vi "Get Object Metadata.vi"(4 "Region":T1, 6 "Version ID":string, 7 "Request Parameters":T2, 8 "error in (no error)":errorcluster, 9 "Bucket":string, 10 "Object Path":string) -> (0 "error out":errorcluster, 2 "HeadObjectResult":T4)   [LabVIEW 2015, in "LV Interface for Amazon S3.lvlib"]
doc: "This operation <B>retrieves information and metadata associated with an object</B> from Amazon S3. You <B>must have READ access</B> to the object. If you grant READ access to the anonymous user, you can return the object without using an authorization header."
uses:
  LV Interface for Amazon S3.lvlib
  Typedefs/AMZ_S3_API_HEADObjectResult.ctl
  Typedefs/AMZ_S3_API_GETObjectResult.ctl
  Typedefs/AMZ_S3_Key-Value pair.ctl
  Typedefs/AMZ_S3_API_GET Object Request Parameters.ctl
  Typedefs/AMZ_S3_API_GET Request Range.ctl
  Typedefs/AMZ_S3_LocationConstraint.ctl
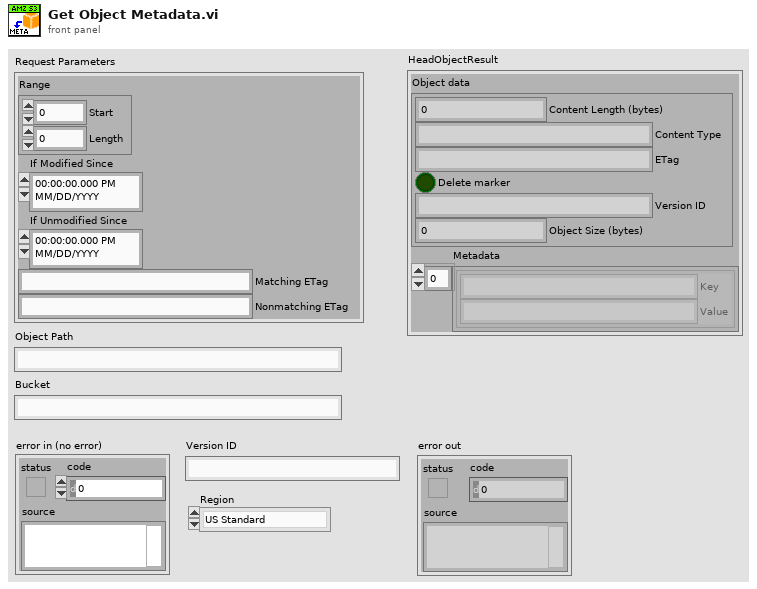
[diagram p1: front panel]
types:
  T1 = typedef "LV Interface for Amazon S3.lvlib/AMZ_S3_LocationConstraint.ctl" = enum16{"US Standard", "us-east-2", "us-west-1", "us-west-2", "ap-northeast-1", "ap-northeast-2", "ap-southeast-1", "ap-southeast-2", "ca-central-1", "eu-central-1", "eu-west-1", "eu-west-2", "sa-east-1"}
  T2 = typedef "LV Interface for Amazon S3.lvlib/AMZ_S3_API_GET Object Request Parameters.ctl" = cluster{"Range":T3, "If Modified Since":timestamp, "If Unmodified Since":timestamp, "Matching ETag":string, "Nonmatching ETag":string}
  T3 = typedef "LV Interface for Amazon S3.lvlib/AMZ_S3_API_GET Request Range.ctl" = cluster{"Start":i64, "Length":i64}
  T4 = typedef "LV Interface for Amazon S3.lvlib/AMZ_S3_API_HEADObjectResult.ctl" = cluster{"Object data":T5, "Metadata":T6[]}
  T5 = typedef "LV Interface for Amazon S3.lvlib/AMZ_S3_API_GETObjectResult.ctl" = cluster{"Content Length (bytes)":u64, "Content Type":string, "ETag":string, "Delete marker":bool, "Version ID":string, "Object Size (bytes)":u64}
  T6 = typedef "LV Interface for Amazon S3.lvlib/AMZ_S3_Key-Value pair.ctl" = cluster{"Key":string, "Value":string}
  T7 = typedef "LV Interface for Amazon S3.lvlib/AMZ_S3_HTTP Header-Value pair.ctl" = cluster{"Header":string, "Value":string}
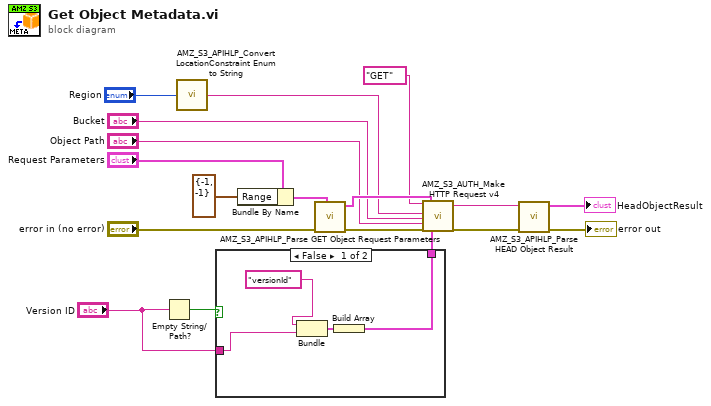
[diagram p0: block diagram]
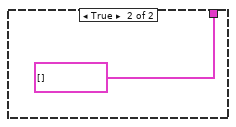
[diagram p2: hidden frame]
diagram:
  n1 = Empty String/Path?(string/path="Version ID") -> (empty?=w5:bool)
  n2 = call "AMZ_S3_APIHLP_Convert LocationConstraint Enum to String.vi"("Location"="Region") -> ("Location String"=w1:string)  [unwired: 4 in]
  n3 = case shown="False" w5 {
    tunnel: [w19 cluster{"item":string, "value":string}[] [] ("request parameters")] -> w3
    tunnel: "Version ID" -> [w22 _]
    frame False {
      n4 = Bundle("versionId", "Version ID"=w22) -> (w20:cluster{string, "Version ID":string})  [unwired: 1 in]
      n5 = Build Array(w20) -> (w19:cluster{string, "Version ID":string}[])
    }
    frame True {
    }
  }
  n6 = Bundle By Name(cluster="Request Parameters", "Range"=T3 {"Start"=-1, "Length"=-1}) -> (w13:T2)
  n7 = call "AMZ_S3_APIHLP_Parse GET Object Request Parameters.vi"("GET Object Request Parameters"=w13, "error in (no error)"="error in (no error)") -> ("error out"=w6:errorcluster, "HTTP Headers"=w10:T7[])  [unwired: 8 in]
  n8 = call "AMZ_S3_AUTH_Make HTTP Request v4.vi"("HTTP-Verb"="GET", "Region"=w1, "Bucket"="Bucket", "Object Key"="Object Path", "error in"=w6, "request headers"=w10, "request parameters"=w3) -> ("response headers"=w11:string, "error out"=w12:errorcluster)  [unwired: 9 in, 2 out]
  n9 = call "AMZ_S3_APIHLP_Parse HEAD Object Result.vi"("error in (no error)"=w12, "Response header"=w11) -> ("error out"=→"error out":errorcluster, "HeadObjectResult"=→"HeadObjectResult":T4)  [unwired: 8 in]
